vi "cam_process_old.vi"(0 "image in":T2) -> (1 "# of red targets":i32, 2 "# of Yellow targets":i32, 3 "# of green targets":i32, 4 "image with hud":T2, 6 "green":cluster{"x-point":dbl, "y-point":dbl}[](array[cluster]), 10 "red":cluster{"x-point":dbl, "y-point":dbl}[](array[cluster]), 15 "yellow":cluster{"x-point":dbl, "y-point":dbl}[](array[cluster]))   [LabVIEW 2018]
uses:
  <vilib>/vision/Image Controls.llb/IMAQ Image.ctl
panel:
  out "Results (Measure 1)":string[][](array[string])
  in  "Tab Control":T1(tab)
  out "XY Graph 2":cluster{dbl[], dbl[]}[](graph)
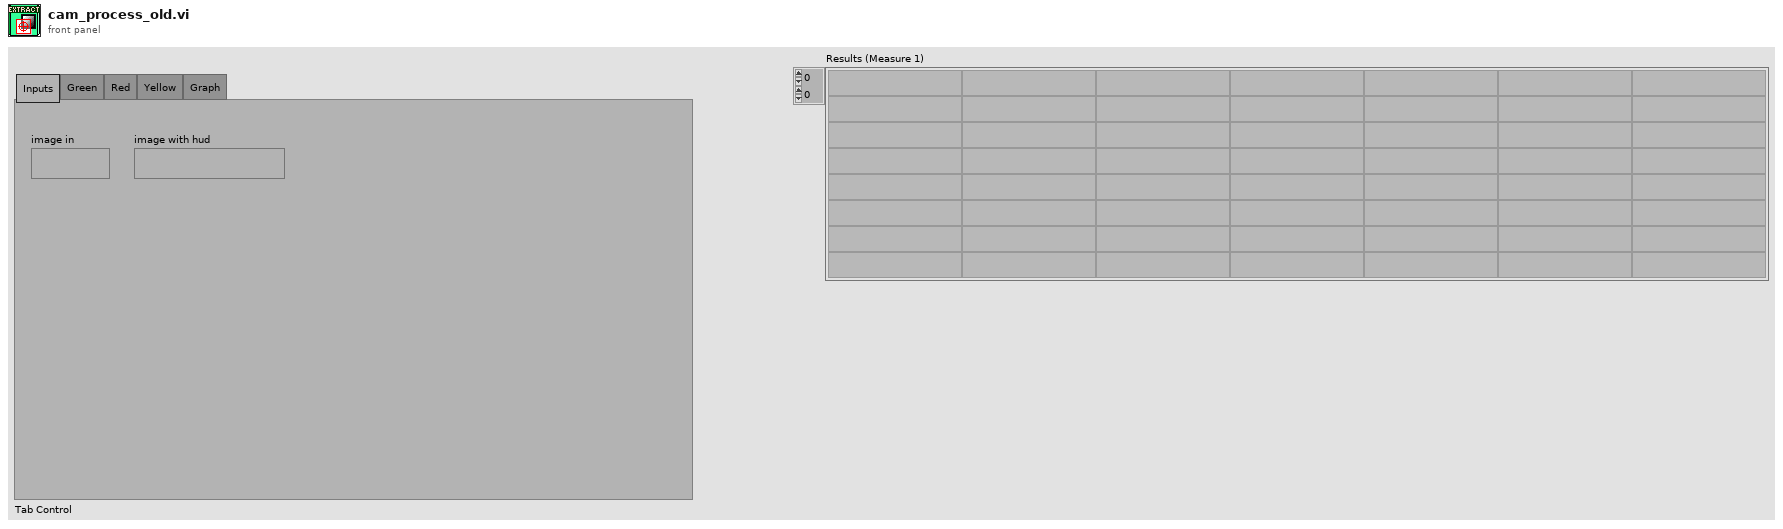
[diagram p1: front panel]
types:
  T1 = enum32{"Inputs", "Green", "Red", "Yellow", "Graph"}
  T2 = typedef "IMAQ Image.ctl" = refnum<image>
  T3 = typedef "Image Type" = u32
  T4 = cluster{"Left":i32, "Top":i32, "Right":i32, "Bottom":i32}
  T5 = cluster{"Particle Measurements (Pixels) (green targets)[0]":dbl, "Particle Measurements (Pixels) (green targets)[1]":dbl, "Particle Measurements (Pixels) (green targets)[2]":dbl, "Particle Measurements (Pixels) (green targets)[3]":dbl, "Particle Measurements (Pixels) (green targets)[4]":dbl, "Particle Measurements (Pixels) (green targets)[5]":dbl, "Particle Measurements (Pixels) (green targets)[6]":dbl, "Particle Measurements (Pixels) (green targets)[7]":dbl, "Particle Measurements (Pixels) (green targets)[8]":dbl}
  T6 = cluster{"Particle Measurements (Pixels) (red targets)[0]":dbl, "Particle Measurements (Pixels) (red targets)[1]":dbl, "Particle Measurements (Pixels) (red targets)[2]":dbl, "Particle Measurements (Pixels) (red targets)[3]":dbl, "Particle Measurements (Pixels) (red targets)[4]":dbl, "Particle Measurements (Pixels) (red targets)[5]":dbl, "Particle Measurements (Pixels) (red targets)[6]":dbl, "Particle Measurements (Pixels) (red targets)[7]":dbl, "Particle Measurements (Pixels) (red targets)[8]":dbl}
  T7 = cluster{"Particle Measurements (Pixels) (Yellow targets)[0]":dbl, "Particle Measurements (Pixels) (Yellow targets)[1]":dbl, "Particle Measurements (Pixels) (Yellow targets)[2]":dbl, "Particle Measurements (Pixels) (Yellow targets)[3]":dbl, "Particle Measurements (Pixels) (Yellow targets)[4]":dbl, "Particle Measurements (Pixels) (Yellow targets)[5]":dbl, "Particle Measurements (Pixels) (Yellow targets)[6]":dbl, "Particle Measurements (Pixels) (Yellow targets)[7]":dbl, "Particle Measurements (Pixels) (Yellow targets)[8]":dbl}
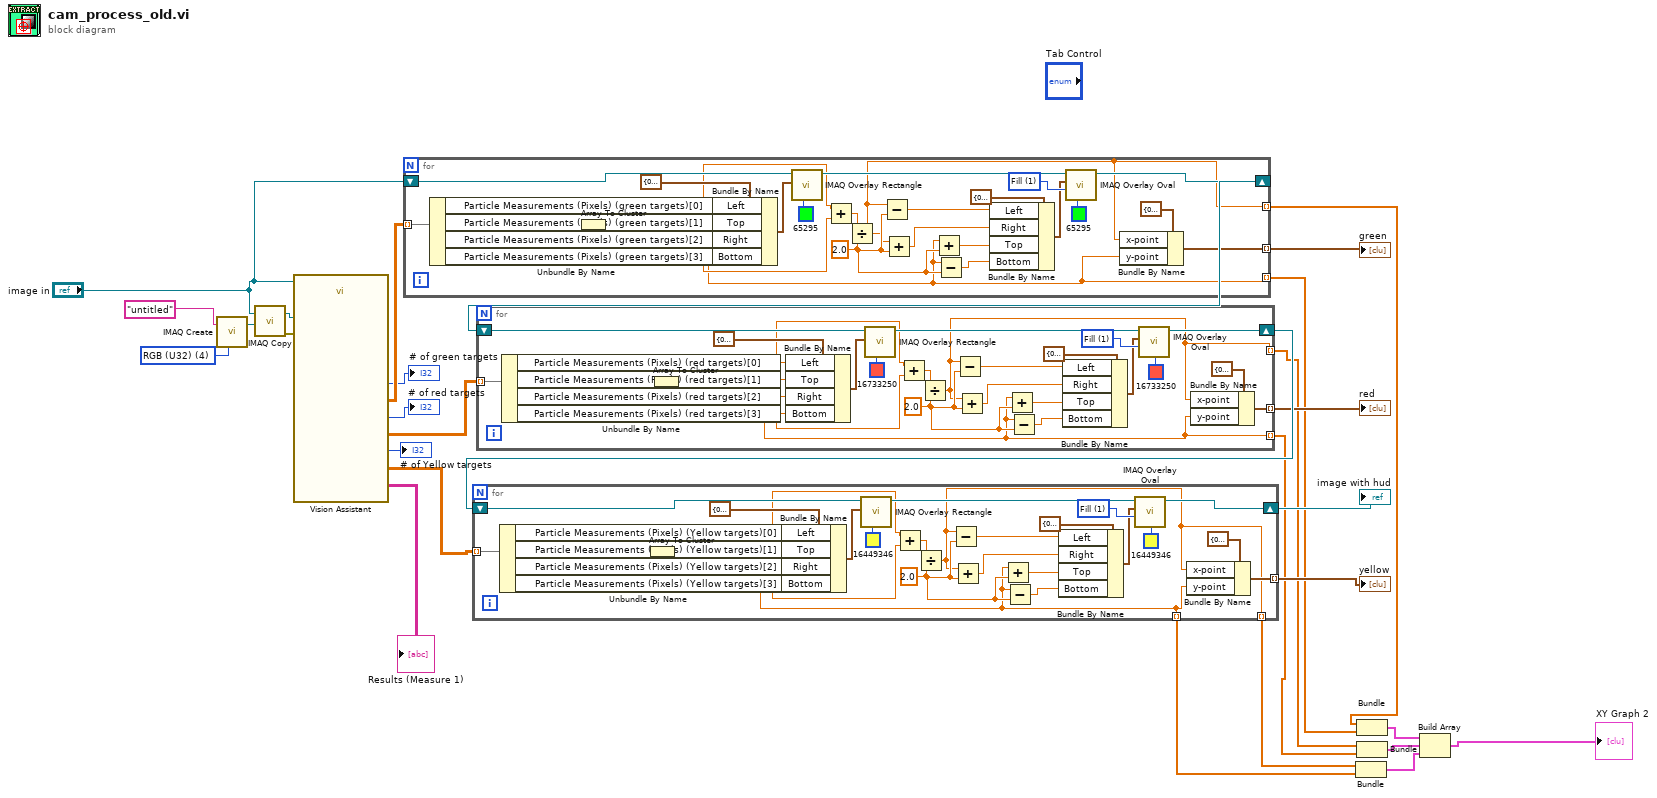
[diagram p0: block diagram]
diagram:
  w25 = T3 4 items=["Grayscale (U8)", "Grayscale (I16)", "Grayscale (SGL)", "Complex (CSG)", "RGB (U32)", "HSL (U32)", "RGB (U64)", "Grayscale (U16)"] ("Image Type")
  n1 = call "IMAQ Create"("Image Name"="untitled", "Image Type"=w25) -> ("New Image"=w15:T2)  [unwired: 3 in, 1 out]
  n2 = call "IMAQ Copy"("Image Dst"=w15, "Image Src"="image in") -> ("error out"=w26:errorcluster, "Image Dst Out"=w17:T2)  [unwired: 4 in]
  n3 = call "Vision Assistant"("Image In"="image in", "Image Dst"=w17, "error in"=w26) -> ("Results (Measure 1)"=→"Results (Measure 1)":string[][], "Number of Particles (green targets)"=→"# of green targets":i32, "Particle Measurements (Pixels) (green targets)"=w27:dbl[][], "Number of Particles (red targets)"=→"# of red targets":i32, "Particle Measurements (Pixels) (red targets)"=w29:dbl[][], "Number of Particles (Yellow targets)"=→"# of Yellow targets":i32, "Particle Measurements (Pixels) (Yellow targets)"=w21:dbl[][])  [unwired: 16 in, 2 out]
  n4 = for {
    tunnel: w27 -> [w51] mode=indexing
    shift-right: [w32] -> w28
    shift-left: "image in" -> [w54]
    tunnel: [w33] -> w12 mode=indexing
    tunnel: [w31] -> w11 mode=indexing
    tunnel: [w30] -> w10 mode=indexing
    w38 = 2.0 ("y")
    w46 = u32 1 items=["Frame", "Fill"] ("Drawing Mode (Frame)")
    n5 = Array To Cluster(array=w51) -> (cluster=w50:T5)
    n6 = Unbundle By Name(w50) -> ("Particle Measurements (Pixels) (green targets)[0]"=w42:dbl, "Particle Measurements (Pixels) (green targets)[1]"=w49:dbl, "Particle Measurements (Pixels) (green targets)[2]"=w41:dbl, "Particle Measurements (Pixels) (green targets)[3]"=w30:dbl)
    n7 = Bundle By Name(cluster=T4 {"Left"=0, "Top"=0, "Right"=0, "Bottom"=0} ("Rectangle"), "Left"=w42, "Top"=w49, "Right"=w41, "Bottom"=w30) -> (w52:T4)
    n8 = call "IMAQ Overlay Rectangle"("Color"=u32 65295, "Rectangle"=w52, "Image"=w54) -> ("Image Out"=w47:T2)  [unwired: 7 in, 1 out]
    n9 = Add(x=w42, y=w41) -> (x+y=w43:dbl)
    n10 = Divide(x=w43, y=w38) -> (x/y=w31:dbl)
    n11 = Subtract(x=w31, y=w38) -> (x-y=w40:dbl)
    n12 = Add(x=w31, y=w38) -> (x+y=w39:dbl)
    n13 = Add(x=w30, y=w38) -> (x+y=w37:dbl)
    n14 = Subtract(x=w30, y=w38) -> (x-y=w36:dbl)
    n15 = Bundle By Name(cluster=T4 {"Left"=0, "Top"=0, "Right"=0, "Bottom"=0} ("Bounding Rectangle"), "Left"=w40, "Right"=w39, "Top"=w37, "Bottom"=w36) -> (w45:T4)
    n16 = call "IMAQ Overlay Oval"("Color"=u32 65295, "Drawing Mode (Frame)"=w46, "Bounding Rectangle"=w45, "Image"=w47) -> ("Image Out"=w32:T2)  [unwired: 6 in, 1 out]
    n17 = Bundle By Name(cluster=cluster{"x-point":dbl, "y-point":dbl} {"x-point"=0.0, "y-point"=0.0} ("input cluster"), "x-point"=w31, "y-point"=w30) -> (w33:cluster{"x-point":dbl, "y-point":dbl})
  }
  "green" <- w12
  n18 = for {
    tunnel: w29 -> [w76] mode=indexing
    shift-right: [w57] -> w18
    shift-left: w28 -> [w79]
    tunnel: [w58] -> w14 mode=indexing
    tunnel: [w56] -> w7 mode=indexing
    tunnel: [w55] -> w6 mode=indexing
    w64 = 2.0 ("y")
    w72 = u32 1 items=["Frame", "Fill"] ("Drawing Mode (Frame)")
    n19 = Array To Cluster(array=w76) -> (cluster=w75:T6)
    n20 = Unbundle By Name(w75) -> ("Particle Measurements (Pixels) (red targets)[0]"=w68:dbl, "Particle Measurements (Pixels) (red targets)[1]"=w74:dbl, "Particle Measurements (Pixels) (red targets)[2]"=w67:dbl, "Particle Measurements (Pixels) (red targets)[3]"=w55:dbl)
    n21 = Bundle By Name(cluster=T4 {"Left"=0, "Top"=0, "Right"=0, "Bottom"=0} ("Rectangle"), "Left"=w68, "Top"=w74, "Right"=w67, "Bottom"=w55) -> (w77:T4)
    n22 = call "IMAQ Overlay Rectangle"("Color"=u32 16733250, "Rectangle"=w77, "Image"=w79) -> ("Image Out"=w73:T2)  [unwired: 7 in, 1 out]
    n23 = Add(x=w68, y=w67) -> (x+y=w69:dbl)
    n24 = Divide(x=w69, y=w64) -> (x/y=w56:dbl)
    n25 = Subtract(x=w56, y=w64) -> (x-y=w66:dbl)
    n26 = Add(x=w56, y=w64) -> (x+y=w65:dbl)
    n27 = Add(x=w55, y=w64) -> (x+y=w63:dbl)
    n28 = Subtract(x=w55, y=w64) -> (x-y=w62:dbl)
    n29 = Bundle By Name(cluster=T4 {"Left"=0, "Top"=0, "Right"=0, "Bottom"=0} ("Bounding Rectangle"), "Left"=w66, "Right"=w65, "Top"=w63, "Bottom"=w62) -> (w71:T4)
    n30 = call "IMAQ Overlay Oval"("Color"=u32 16733250, "Drawing Mode (Frame)"=w72, "Bounding Rectangle"=w71, "Image"=w73) -> ("Image Out"=w57:T2)  [unwired: 6 in, 1 out]
    n31 = Bundle By Name(cluster=cluster{"x-point":dbl, "y-point":dbl} {"x-point"=0.0, "y-point"=0.0} ("input cluster"), "x-point"=w56, "y-point"=w55) -> (w58:cluster{"x-point":dbl, "y-point":dbl})
  }
  "red" <- w14
  n32 = for {
    tunnel: w21 -> [w101] mode=indexing
    shift-right: [w97] -> w20
    shift-left: w18 -> [w104]
    tunnel: [w82] -> w13 mode=indexing
    tunnel: [w81] -> w3 mode=indexing
    tunnel: [w80] -> w2 mode=indexing
    w88 = 2.0 ("y")
    w96 = u32 1 items=["Frame", "Fill"] ("Drawing Mode (Frame)")
    n33 = Array To Cluster(array=w101) -> (cluster=w100:T7)
    n34 = Unbundle By Name(w100) -> ("Particle Measurements (Pixels) (Yellow targets)[0]"=w92:dbl, "Particle Measurements (Pixels) (Yellow targets)[1]"=w99:dbl, "Particle Measurements (Pixels) (Yellow targets)[2]"=w91:dbl, "Particle Measurements (Pixels) (Yellow targets)[3]"=w80:dbl)
    n35 = Bundle By Name(cluster=T4 {"Left"=0, "Top"=0, "Right"=0, "Bottom"=0} ("Rectangle"), "Left"=w92, "Top"=w99, "Right"=w91, "Bottom"=w80) -> (w102:T4)
    n36 = call "IMAQ Overlay Rectangle"("Color"=u32 16449346, "Rectangle"=w102, "Image"=w104) -> ("Image Out"=w98:T2)  [unwired: 7 in, 1 out]
    n37 = Add(x=w92, y=w91) -> (x+y=w93:dbl)
    n38 = Divide(x=w93, y=w88) -> (x/y=w81:dbl)
    n39 = Subtract(x=w81, y=w88) -> (x-y=w90:dbl)
    n40 = Add(x=w81, y=w88) -> (x+y=w89:dbl)
    n41 = Add(x=w80, y=w88) -> (x+y=w87:dbl)
    n42 = Subtract(x=w80, y=w88) -> (x-y=w86:dbl)
    n43 = Bundle By Name(cluster=T4 {"Left"=0, "Top"=0, "Right"=0, "Bottom"=0} ("Bounding Rectangle"), "Left"=w90, "Right"=w89, "Top"=w87, "Bottom"=w86) -> (w95:T4)
    n44 = call "IMAQ Overlay Oval"("Color"=u32 16449346, "Drawing Mode (Frame)"=w96, "Bounding Rectangle"=w95, "Image"=w98) -> ("Image Out"=w97:T2)  [unwired: 6 in, 1 out]
    n45 = Bundle By Name(cluster=cluster{"x-point":dbl, "y-point":dbl} {"x-point"=0.0, "y-point"=0.0} ("input cluster"), "x-point"=w81, "y-point"=w80) -> (w82:cluster{"x-point":dbl, "y-point":dbl})
  }
  "image with hud" <- w20
  "yellow" <- w13
  n46 = Bundle(w3, w2) -> (w4:cluster{dbl[], dbl[]})  [unwired: 1 in]
  n47 = Bundle(w11, w10) -> (w9:cluster{dbl[], dbl[]})  [unwired: 1 in]
  n48 = Bundle(w7, w6) -> (w5:cluster{dbl[], dbl[]})  [unwired: 1 in]
  n49 = Build Array(w9, w5, w4) -> (→"XY Graph 2":cluster{dbl[], dbl[]}[])
